vi "save_log.vi"() -> ()   [LabVIEW 2024]
panel:
  in  "错误输入":errorcluster
  out "错误输出":errorcluster
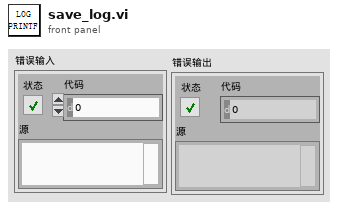
[diagram p1: front panel]
types:
  T1 = enum16{"open", "replace", "create", "open or create", "replace or create", "replace or create with confirmation"}
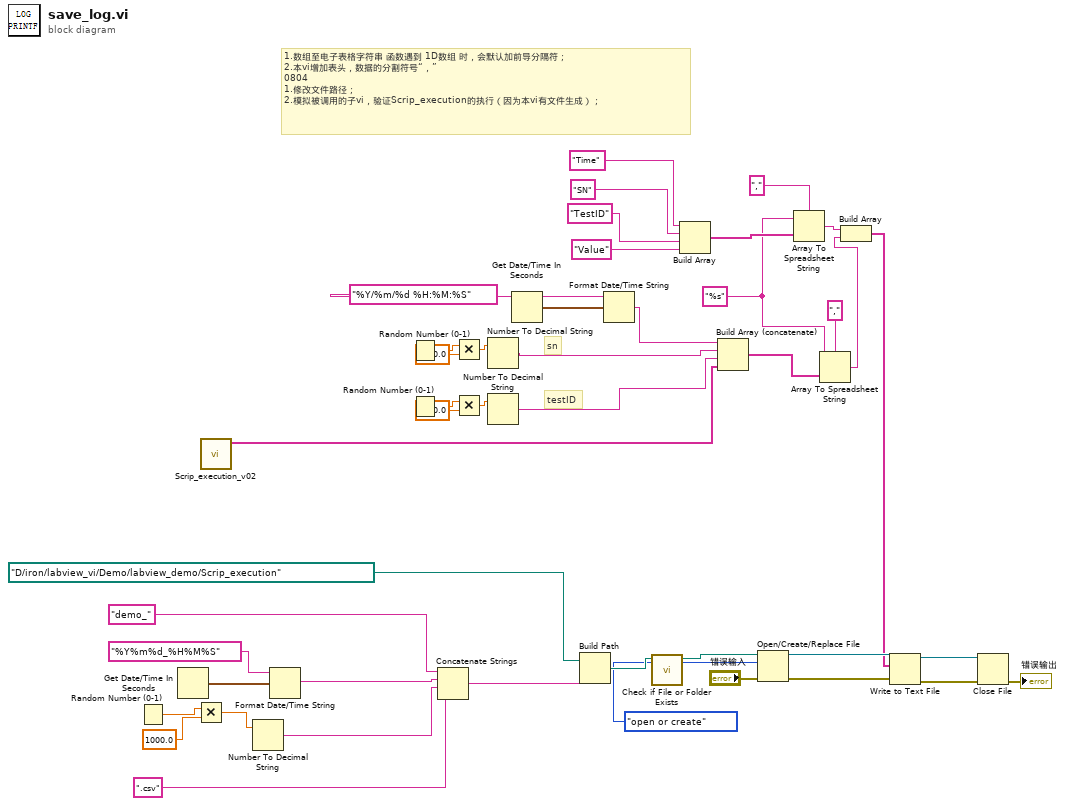
[diagram p0: block diagram]
diagram:
  w23 = "%s" ("格式字符串")
  # "testID"
  # "sn"
  # "1.数组至电子表格字符串 函数遇到 1D数组 时，会默认加前导分隔符；\n2.本vi增加表头，数据的分割符号“，”\n0804\n1.修改文件路径；\n2.模拟被调用的子vi，验证Scrip_execution的执行（因为本vi有文件生成）；"
  n1 = Random Number (0-1)() -> (number: 0 to 1=w6:dbl)
  n2 = Get Date/Time In Seconds() -> (seconds since 1Jan1904=w32:timestamp)
  n3 = Multiply(x=w6, y=1000.0) -> (x*y=w4:dbl)
  n4 = call "Scrip_execution_v02.vi"() -> ("添加的数组"=w1:string[])  [unwired: 11 in]
  n5 = Number To Decimal String(number=w4) -> (decimal integer string=w3:string)  [unwired: 1 in]
  n6 = Format Date/Time String(time format string (%c)="%Y%m%d_%H%M%S" ("时间格式字符串(%c)"), seconds (now)=w32) -> (date/time string=w31:string)  [unwired: 1 in]
  n7 = Random Number (0-1)() -> (number: 0 to 1=w18:dbl)
  n8 = Random Number (0-1)() -> (number: 0 to 1=w12:dbl)
  n9 = Concatenate Strings("demo_" ("字符串"), w31, w3, ".csv" ("字符串")) -> (w34:string)
  n10 = Multiply(x=w18, y=1000.0) -> (x*y=w16:dbl)
  n11 = Multiply(x=w12, y=1000.0) -> (x*y=w14:dbl)
  n12 = Number To Decimal String(number=w16) -> (decimal integer string=w15:string)  [unwired: 1 in]
  n13 = Number To Decimal String(number=w14) -> (decimal integer string=w11:string)  [unwired: 1 in]
  n14 = Get Date/Time In Seconds() -> (seconds since 1Jan1904=w42:timestamp)
  n15 = Build Path(base path=path "D:/iron/labview_vi/Demo/labview_demo/Scrip_execution" ("基路径"), name or relative path=w34) -> (appended path=w44:path)
  n16 = Format Date/Time String(time format string (%c)="%Y/%m/%d %H:%M:%S" ("时间格式字符串(%c)"), seconds (now)=w42) -> (date/time string=w30:string)  [unwired: 1 in]
  n17 = call <vilib>:"Check if File or Folder Exists.vi"("path"=w44) -> ("dup path"=w43:path)  [unwired: 8 in, 2 out]
  n18 = Build Array("Time" ("元素"), "SN" ("元素"), "TestID" ("元素"), "Value" ("元素")) -> (w24:string[])
  n19 = Build Array (concatenate)(w30, w15, w11, w1) -> (w40:string[])
  n20 = Open/Create/Replace File(file path (use dialog)=w43, error in="错误输入", operation (0:open)=T1."open or create" ("操作(0:open)")) -> (refnum out=w38:refnum<file>, error out=w10:errorcluster)  [unwired: 3 in, 1 out]
  n21 = Array To Spreadsheet String(delimiter (Tab)="," ("分隔符(Tab)"), array=w24, 3:w23) -> (spreadsheet string=w21:string)
  n22 = Array To Spreadsheet String(delimiter (Tab)="," ("分隔符(Tab)"), array=w40, 3:w23) -> (spreadsheet string=w20:string)
  n23 = Build Array(w21, w20) -> (w19:string[])
  n24 = Write to Text File(file (use dialog)=w38, text=w19, error in=w10) -> (refnum out=w37:refnum<file>, error out=w9:errorcluster)  [unwired: 1 in, 1 out]
  n25 = Close File(refnum=w37, error in=w9) -> (error out=→"错误输出":errorcluster)  [unwired: 1 out]
